vi "Append Paragraph with Link.vi"(0 "PDF Report":T24(xcontrol), 2 "Text":T2={"Text"={"Text"="", "Font"={"Name"="", "Size"=-1.0, "Color"=0, "Style"={"Bold"=FALSE, "Italic"=FALSE, "Underline"=FALSE, "Strikeout"=FALSE}}}, "Link"={"Hyperlink"="", "Font"={"Name"="", "Size"=-1.0, "Color"=255, "Style"={"Bold"=FALSE, "Italic"=TRUE, "Underline"=FALSE, "Strikeout"=FALSE}}}, "Paragraphe"={" Aligment"=enum."Select", "Line spacing"=enum."Select"}, "Indentation"={"Left"=0.0, "Right"=0.0}}, 11 "error in (no error)":errorcluster, 13 "Image to Add refnum [ ]":T1) -> (4 "PDF Report duplicate":T24(xcontrol), 15 "error out":errorcluster)   [LabVIEW 2013]
doc: "Appends text with a <B>line feed</B>, at the end, to the PDF report. This text can be <B>aligned</B> (CENTER, JUSTIFY, LEFT, RIGHT) and <B>indented</B>. \n\nIf <B>Font</B> and <B>Pararaph properties</B> are not specified then the <B>Default font</B> and <B>Default paragraph</B> will be use.\n\nThe data type you wire to the <B>Text</B> input determines the polymorphic instance to use.\n\n<B>FRANÇAIS</B>\nAjoute au rapport PDF du texte sous la forme d'un paragraphe terminé avec un \"<B>Line Feed</B>\". Ce texte peut être <B>aligné</B> (CENTER, JUSTIFY, LEFT, RIGHT) et avoir un <B>renfoncement</B> (gauche et droit) pour tout le paragraphe.\n\nSi la police de caractères <B>Font</B> et les propriétés <B>Pararaph properties</B> ne sont pas spécifiés alors la police par défaut <B>Default font</B> et <B>Default paragraph</B> seront utilisées.\n\nLe type de données que vous connectez au terminal <B>Text</B> détermine l'instance polymorphique utilisée.\n\nVersion 1.0\nDeveloped by Jean-Marc Simard\nCopyright © 2010, Exaprom Inc.\nAll rights reserved.\nLicense: BSD\n\nWith iTextSharp 4.1.6 (http://itextsharp.sourceforge.net)\nunder Mozilla Public License Version 1.1\n(http://www.mozilla.org/MPL/MPL-1.1.html)"
uses:
  Controls/PDF Report Xcontrol/PDF Report.xctl
  Controls/Text and hyperlink.ctl
  Controls/Font cluster.ctl
  Controls/Font size.ctl
  Controls/Font color.ctl
  Controls/Paragraphe cluster.ctl
  Controls/Texte alignement.ctl
  Controls/Line spacing.ctl
  Controls/Paragraph indentation.ctl
  Controls/Image to Add refnum [ ].ctl
  C:/Users/MaxCorp/Documents/GitHub/TopView/DLL/itextsharp.dll
  DLL/itextsharp.dll
  Controls/Phrase or paragraph.ctl
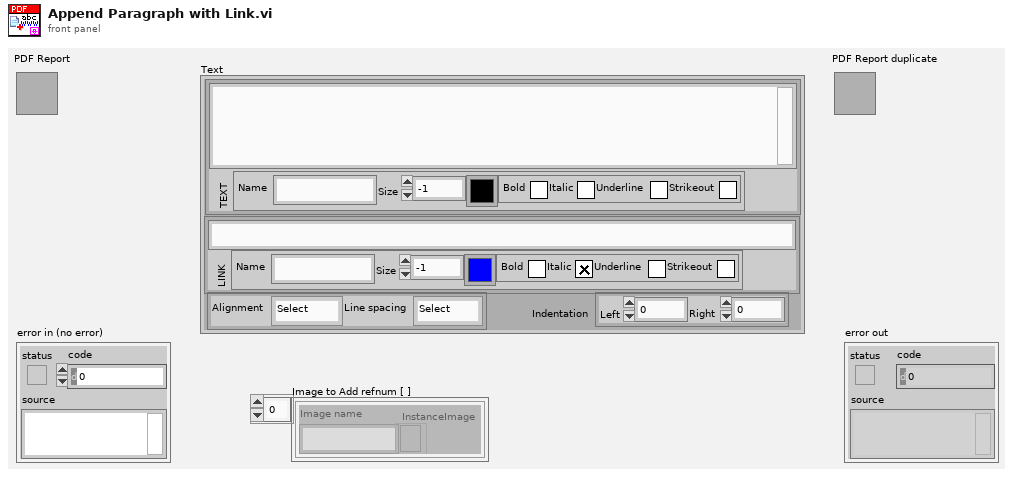
[diagram p1: front panel]
types:
  T1 = typedef "Image to Add refnum [ ].ctl" = cluster{"Image name":string, "InstanceImage":refnum<k24>}[]
  T2 = typedef "Text and hyperlink.ctl" = cluster{"Text":cluster{"Text":string, "Font":T3}, "Link":cluster{"Hyperlink":string, "Font":T3}, "Paragraphe":T6, "Indentation":T9}
  T3 = typedef "Font cluster.ctl" = cluster{"Name":string, "Size":T4, "Color":T5, "Style":cluster{"Bold":bool, "Italic":bool, "Underline":bool, "Strikeout":bool}}
  T4 = typedef "Font size.ctl" = sgl
  T5 = typedef "Font color.ctl" = u32
  T6 = typedef "Paragraphe cluster.ctl" = cluster{" Aligment":T7, "Line spacing":T8}
  T7 = typedef "Texte alignement.ctl" = enum16{"Select", "CENTER", "JUSTIFY", "LEFT", "RIGHT"}
  T8 = typedef "Line spacing.ctl" = enum16{"Select", "1.0", "1.5", "2.0"}
  T9 = typedef "Paragraph indentation.ctl" = cluster{"Left":sgl, "Right":sgl}
  T10 = typedef "Unit.ctl" = enum16{"inch", "mm"}
  T11 = typedef "Page dimensions.ctl" = cluster{"Start at page":i32, "Orientation":T12, "widht":sgl, "height":sgl, "Margin left":sgl, "Margin right":sgl, "Margin top":sgl, "Margin bottom":sgl}
  T12 = typedef "Page Orientation.ctl" = enum16{"Portrait", "Landscape"}
  T13 = typedef "Image or Table Caption.ctl" = cluster{"Caption":string, "Separator":string, "Position":enum16{"Above", "Below"}}
  T14 = typedef "Header Footer [ ].ctl" = T15[]
  T15 = typedef "Header Footer cluster.ctl" = cluster{"Start page":i32, "Type":T16, "Alignment":T17, "Vertical Alignement":T18, "Image (%)":sgl, "Page #":T19, "Text":string, "Path":string, "Font":T3, "Font refnum":refnum<k24>, "Line":cluster{"Line":T20, "Thickness (points)":sgl, "Colour":T5}}
  T16 = typedef "Header Footer Type.ctl" = enum16{"Select", "Text", "Text + hyperlink", "Page number", "Image", "Image + hyperlink"}
  T17 = typedef "Header footer horiz alignment.ctl" = enum16{"Left", "Center", "Right"}
  T18 = typedef "Cell Vertical alignment.ctl" = enum16{"TOP", "MIDDLE", "BOTTOM"}
  T19 = typedef "Page number.ctl" = cluster{"Text 1":string, "Text 2":string, "Text 3":string}
  T20 = typedef "Header Footer Line.ctl" = enum16{"No line", "Horizontal line"}
  T21 = typedef "Watermark cluster2.ctl" = cluster{"Show? (F)":bool, "Type":enum16{"Image", "Text"}, "Opacity (%)":sgl, "Rotate(°)":sgl, "Position":cluster{"Position":T22, "X":sgl, "Y":sgl}, "Image path":path, "Scaled(%)":sgl, "Image refnum":refnum<k24>, "Text":string, "Font":cluster{"Name":string, "Size":T4, "Color":T5}, "Font refnum":refnum<k24>, "Alignment":T17, "Automatic":bool}
  T22 = typedef "Watermark Position.ctl" = enum16{"Absolute", "Center (page)", "Center (text section)"}
  T23 = typedef "System Fonts.ctl" = cluster{"Font name [ ]":string[], "Font and file names [ ]":cluster{"Font name":string, "File name":string}[]}
  T24 = cluster{"Document":refnum<k24>, "Writer":refnum<k24>, "Default Font":refnum<k24>, "Default Font cluster":T3, "Path":path, "Unit (default = mm)":T10, "Paragraphe cluster":T6, "Pages dimensions [ ]":T11[], "Captions":cluster{"Image":T13, "Image counter":u16, "Table":T13, "Table counter":u16, "Font":T3}, "Header":T14, "Footer":T14, "Watermark ":T21, "Actual VI name":string, "System Fonts":T23}
  T25 = typedef "Phrase or paragraph.ctl" = enum16{"Add to Phrase", "Add to Paragraph", "Create Phrase", "Create Paragraph"}
  T26 = typedef "Text type.ctl" = enum16{"empty", "Text", "Hyperlink"}
  T27 = cluster{"Text type":T26, "Text":string, "Hyperlink":string}[]
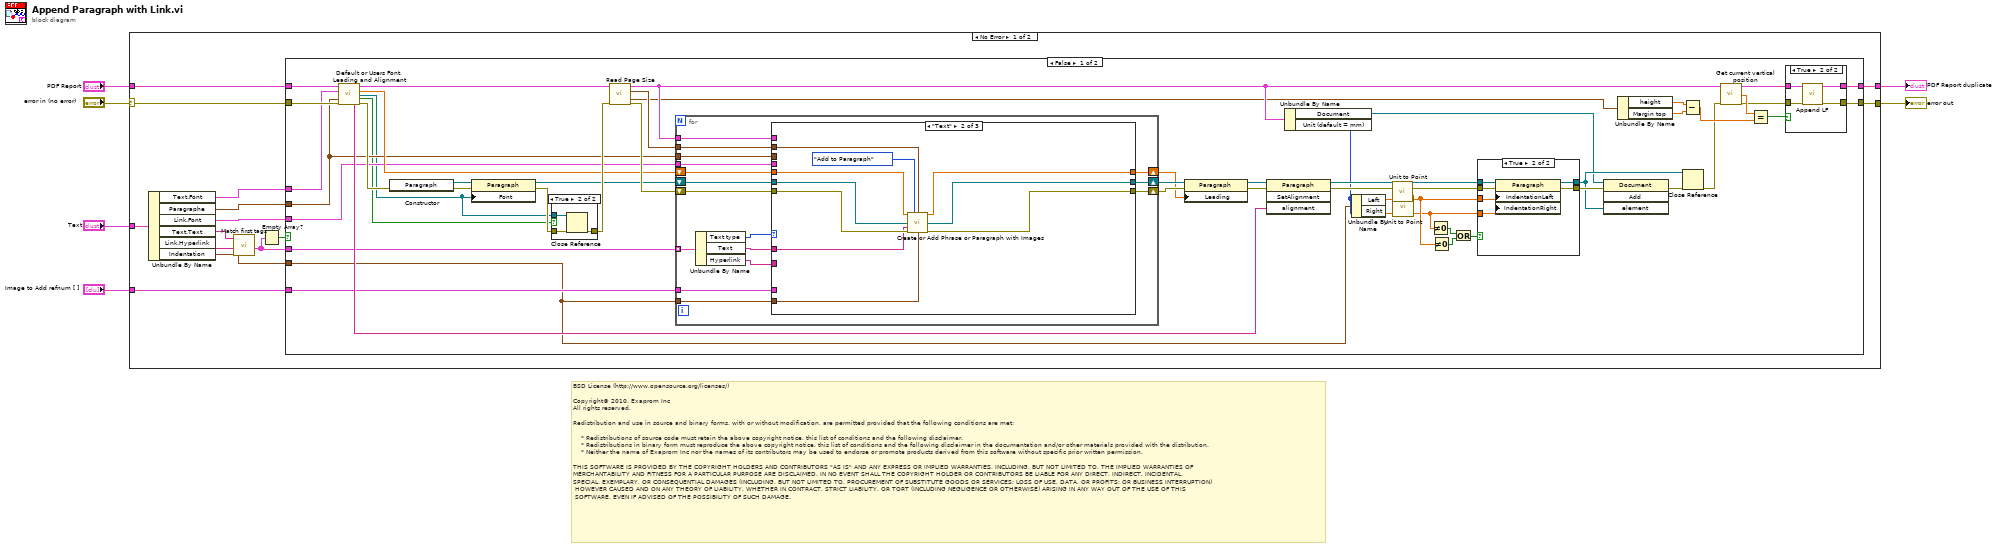
[diagram p0: block diagram]
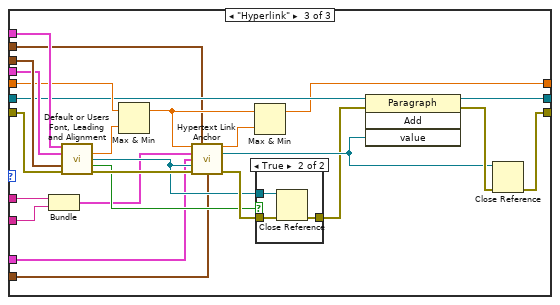
[diagram p4: hidden frame]
diagram:
  # "BSD License (http://www.opensource.org/licenses/)\n\nCopyright© 2010, Exaprom Inc\nAll rights reserved.\n\nRedistribution and use in source and binary forms, with or without modification, are permitted provided that the following conditions are met:\n\n    * Redistributions of source code must retain the above copyright notice, this list of conditions and the following disclaimer.\n    * Redistributions in binary form must reproduce the above copyright notice, this list of conditions and the following disclaimer in the documentation and/or other materials provided with the distribution.\n    * Neither the name of Exaprom Inc nor the names of its contributors may be used to endorse or promote products derived from this software without specific prior written permission.\n\nTHIS SOFTWARE IS PROVIDED BY THE COPYRIGHT HOLDERS AND CONTRIBUTORS \"AS IS\" AND ANY EXPRESS OR IMPLIED WARRANTIES, INCLUDING, BUT NOT LIMITED TO, THE IMPLIED WARRANTIES OF \nMERCHANTABILITY AND FITNESS FOR A PARTICULAR PURPOSE ARE DISCLAIMED. IN NO EVENT SHALL THE COPYRIGHT HOLDER OR CONTRIBUTORS BE LIABLE FOR ANY DIRECT, INDIRECT, INCIDENTAL,\nSPECIAL, EXEMPLARY, OR CONSEQUENTIAL DAMAGES (INCLUDING, BUT NOT LIMITED TO, PROCUREMENT OF SUBSTITUTE GOODS OR SERVICES; LOSS OF USE, DATA, OR PROFITS; OR BUSINESS INTERRUPTION)\n HOWEVER CAUSED AND ON ANY THEORY OF LIABILITY, WHETHER IN CONTRACT, STRICT LIABILITY, OR TORT (INCLUDING NEGLIGENCE OR OTHERWISE) ARISING IN ANY WAY OUT OF THE USE OF THIS\n SOFTWARE, EVEN IF ADVISED OF THE POSSIBILITY OF SUCH DAMAGE."
  n1 = case shown="No Error" "error in (no error)" {
    selector: "error in (no error)" -> [w15 w152]
    tunnel: [w17 w152] -> w6
    tunnel: "PDF Report" -> [w16 w151]
    tunnel: [w18 w151] -> w3
    tunnel: "Text" -> [w20 _]
    tunnel: "Image to Add refnum [ ]" -> [w13 _]
    frame No Error {
      n2 = Unbundle By Name(w20) -> ("Text.Font"=w9:T3, "Paragraphe"=w12:T6, "Link.Font"=w7:T3, "Text.Text"=w8:string, "Link.Hyperlink"=w14:string, "Indentation"=w19:T9)
      n3 = call "Match first tags.vi"("Hyperlink"=w14, "Text"=w8) -> ("Array"=w10:T27)  [unwired: 2 in, 7 out]
      n4 = Empty Array?(array=w10) -> (empty?=w11:bool)
      n5 = case shown="False" w11 {
        tunnel: w19 -> [w30 _]
        tunnel: [w46 w150] -> w18
        tunnel: [w44 w149] -> w17
        tunnel: w9 -> [w42 _]
        tunnel: w16 -> [w26 w150]
        tunnel: w15 -> [w68 w149]
        tunnel: w10 -> [w36 _]
        tunnel: w13 -> [w33 _]
        tunnel: w12 -> [w32 _]
        tunnel: w7 -> [w25 _]
        frame False {
          n6 = call "Default or Users Font, Leading and Alignment.vi"("PDF Report"=w26, "Font"=w42, "Paragraphe cluster"=w32, "error in (no error)"=w68) -> ("PDF Report duplicate"=w28:T24, "Leading"=w35:T4, "Font Ref"=w22:refnum<k24>, "Close Font Ref"=w21:bool, "Aligment"=w67:string, "error out"=w69:errorcluster)  [unwired: 6 out]
          n7 = constructor class="Paragraph"(error in=w69) -> (reference out=w40:refnum<k24>, error out=w39:errorcluster)  [unwired: 2 in, 1 out]
          n8 = property class="Paragraph"(reference=w40, error in=w39, "Font"=w22) -> (reference out=w38:refnum<k24>, error out=w23:errorcluster)
          n9 = case shown="True" w21 {
            tunnel: [w73 w76] -> w70
            tunnel: w23 -> [w73 w75]
            tunnel: w22 -> [_ w74]
            frame False {
            }
            frame True {
              n10 = Close Reference(reference=w74, error in (no error)=w75) -> (error out=w76:errorcluster)
            }
          }
          n11 = call "Read Page Size.vi"("PDF Report"=w28, "error in (no error)"=w70) -> ("PDF Report duplicate"=w29:T24, "Text zone (points)"=w27:cluster{"widht":sgl, "height":sgl}, "Page (points)"=w24:T11, "error out"=w71:errorcluster)  [unwired: 10 out]
          n12 = for {
            tunnel: w36 -> [w92] mode=indexing
            shift-right: [w85] -> w72
            shift-left: w71 -> [w91]
            shift-right: [w88] -> w37
            shift-left: w38 -> [w89]
            shift-right: [w83] -> w34
            shift-left: w35 -> [w84]
            tunnel: w33 -> [w82]
            tunnel: w25 -> [w81]
            tunnel: w32 -> [w80]
            tunnel: w29 -> [w79]
            tunnel: w27 -> [w78]
            tunnel: w30 -> [w77]
            n13 = Unbundle By Name(w92) -> ("Text type"=w90:T26, "Text"=w87:string, "Hyperlink"=w86:string)
            n14 = case shown="\"Text\"" w90 {
              tunnel: [w95 w103 w117] -> w88
              tunnel: w80 -> [_ _ w123]
              tunnel: w81 -> [_ _ w122]
              tunnel: w79 -> [_ _ w121]
              tunnel: w91 -> [w94 w105 w114]
              tunnel: w89 -> [w95 w102 w115]
              tunnel: [w94 w104 w116] -> w85
              tunnel: w82 -> [_ _ w118]
              tunnel: w84 -> [w93 w99 w120]
              tunnel: [w93 w98 w108] -> w83
              tunnel: w87 -> [_ w100 w113]
              tunnel: w86 -> [_ _ w112]
              tunnel: w78 -> [_ w97 w107]
              tunnel: w77 -> [_ w96 w106]
              frame "empty", Default {
              }
              frame "Text" {
                n15 = call "Create or Add Phrase or Paragraph with Images.vi"("Leading"=w99, "Phrase or paragraph"=Phrase_or_paragraph."Add to Paragraph", "Text zone (points)"=w97, "Paragraph refnum IN"=w102, "Text"=w100, "error in (no error)"=w105, "Paragraph indentation (points)"=w96) -> ("Leading duplicate"=w98:sgl, "Paragraph refnum OUT"=w103:refnum<k24>, "error out"=w104:errorcluster)  [unwired: 4 in, 2 out]
              }
              frame "Hyperlink" {
                n16 = Bundle("Text"=w113, "Hyperlink"=w112) -> (w111:cluster{"Text":string, "Hyperlink":string})  [unwired: 1 out]
                n17 = call "Default or Users Font, Leading and Alignment.vi"("PDF Report"=w121, "Font"=w122, "Paragraphe cluster"=w123, "error in (no error)"=w114) -> ("Leading"=w119:T4, "Font Ref"=w125:refnum<k24>, "Close Font Ref"=w124:bool, "error out"=w128:errorcluster)  [unwired: 8 out]
                n18 = Max & Min(x=w120, y=w119) -> (max(x,y)=w110:T4)  [unwired: 1 out]
                n19 = call "Hypertext Link Anchor.vi"("Leading"=w110, "Text zone (points)"=w107, "Hyperlink"=w111, "Image to Add refnum [ ]"=w118, "Font refnum"=w125, "error in (no error)"=w128, "Paragraph indentation (points)"=w106) -> ("Leading OUT"=w109:sgl, "Anchor"=w129:refnum<k24>, "error out"=w127:errorcluster)  [unwired: 1 in, 5 out]
                n20 = Max & Min(x=w110, y=w109) -> (max(x,y)=w108:T4)  [unwired: 1 out]
                n21 = case shown="True" w124 {
                  tunnel: [w131 w134] -> w126
                  tunnel: w127 -> [w131 w133]
                  tunnel: w125 -> [_ w132]
                  frame False {
                  }
                  frame True {
                    n22 = Close Reference(reference=w132, error in (no error)=w133) -> (error out=w134:errorcluster)
                  }
                }
                n23 = invoke class="Paragraph" method="Add"(reference=w115, error in=w126, "value"=w129) -> (reference out=w117:refnum<k24>, error out=w130:errorcluster)  [unwired: 1 in, 2 out]
                n24 = Close Reference(reference=w129, error in (no error)=w130) -> (error out=w116:errorcluster)
              }
            }
          }
          n25 = property class="Paragraph"(reference=w37, error in=w72, "Leading"=w34) -> (reference out=w41:refnum<k24>, error out=w52:errorcluster)
          n26 = invoke class="Paragraph" method="SetAlignment"(reference=w41, error in=w52, "alignment"=w67) -> (reference out=w57:refnum<k24>, error out=w58:errorcluster)  [unwired: 1 in, 2 out]
          n27 = Unbundle By Name(w29) -> ("Document"=w53:refnum<k24>, "Unit (default = mm)"=w54:T10)
          n28 = Unbundle By Name(w30) -> ("Left"=w62:sgl, "Right"=w63:sgl)
          n29 = call "Unit to Point.vi"("X unit"=w62, "Unit (default = mm)"=w54) -> ("X point"=w56:sgl)  [unwired: 7 out]
          n30 = call "Unit to Point.vi"("X unit"=w63, "Unit (default = mm)"=w54) -> ("X point"=w55:sgl)  [unwired: 7 out]
          n31 = Not Equal To 0?(x=w55) -> (x != 0?=w60:bool)
          n32 = Not Equal To 0?(x=w56) -> (x != 0?=w59:bool)
          n33 = Or(x=w60, y=w59) -> (x .or. y?=w61:bool)
          n34 = case shown="True" w61 {
            tunnel: w57 -> [w142 w148]
            tunnel: w58 -> [w141 w147]
            tunnel: [w141 w146] -> w65
            tunnel: [w142 w145] -> w64
            tunnel: w56 -> [_ w144]
            tunnel: w55 -> [_ w143]
            frame False {
            }
            frame True {
              n35 = property class="Paragraph"(reference=w148, error in=w147, "IndentationLeft"=w144, "IndentationRight"=w143) -> (reference out=w145:refnum<k24>, error out=w146:errorcluster)
            }
          }
          n36 = invoke class="Document" method="Add"(reference=w53, error in=w65, "element"=w64) -> (error out=w66:errorcluster)  [unwired: 1 in, 3 out]
          n37 = Unbundle By Name(w24) -> ("height"=w50:sgl, "Margin top"=w49:sgl)
          n38 = Subtract(x=w50, y=w49) -> (x-y=w47:sgl)
          n39 = Close Reference(reference=w64, error in (no error)=w66) -> (error out=w31:errorcluster)
          n40 = call "Get current vertical position.vi"("PDF Report In"=w29, "error in (no error)"=w31) -> ("PDF Report duplicate"=w51:T24, "GetVerticalPosition (points)"=w48:sgl, "error out"=w45:errorcluster)  [unwired: 1 in, 10 out]
          n41 = Equal?(x=w48, y=w47) -> (x = y?=w43:bool)
          n42 = case shown="True" w43 {
            tunnel: w51 -> [w136 w140]
            tunnel: [w136 w139] -> w46
            tunnel: w45 -> [w135 w138]
            tunnel: [w135 w137] -> w44
            frame False {
            }
            frame True {
              n43 = call "Append LF.vi"("PDF Report IN"=w140, "error in (no error)"=w138) -> ("PDF Report duplicate"=w139:T24, "error out"=w137:errorcluster)  [unwired: 1 in, 11 out]
            }
          }
        }
        frame True {
        }
      }
    }
    frame Error {
    }
  }
  "error out" <- w6
  "PDF Report duplicate" <- w3
